vi "NT Add NullSubscriber.vi"(8 "error in (no error)":errorcluster, 11 "match Pattern":string) -> (0 "error out":errorcluster)   [LabVIEW 2025]
uses:
  FRC_NetworkTablesLV.dll
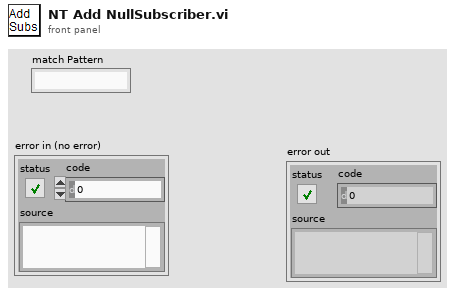
[diagram p1: front panel]
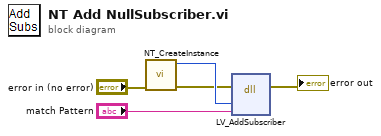
[diagram p0: block diagram]
diagram:
  n1 = call <vilib>:"NT_CreateInstance.vi"("error in (no error)"="error in (no error)") -> ("error out"=w3:errorcluster, "InstanceHandle"=w4:u64)  [unwired: 9 in]
  n2 = dll-call lib="FRC_NetworkTablesLV.*" fn="LV_AddSubscriber"(error in=w3, "inst"=w4, "prefix"="match Pattern") -> (error out=→"error out":errorcluster)  [unwired: 5 in, 1 out]
